vi "Global_Variables.vi"() -> ()   [LabVIEW 2018]
panel:
  in  "Timing Script Wait Tag":string="Wait"
  in  "Max FFT Samples":i32=8000000 min=0 max=8000000
  in  "GraphXY Points per Pixel":i32=800
  in  "Default XML":string="default.xml"
  in  "Running XML":string="running.xml"
  in  "Timing Script Generate Tag":string="Generate"
  in  "Last XML":string="last.xml"
  in  "Timing Script Acq Tag":string="Acq"
  in  "Timing Script Excit Tag":string="Excit"
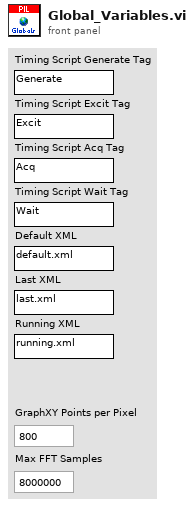
[diagram p1: front panel]
diagram:
